vi "Compute Transfer Rate for FPGA.vi"(6 "Duty Rate":u16, 7 "Clock Rate (minus 1)":u16) -> (2 "Current Value":u16, 3 "Output":bool)   [LabVIEW 2013]
doc: "This SubVI uses a counter to create a boolean output based upon the requested number of clock cycles and a duty cycle."
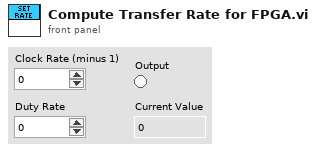
[diagram p1: front panel]
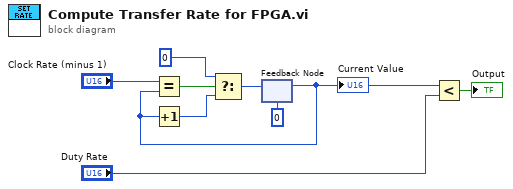
[diagram p0: block diagram]
diagram:
  n1 = feedback #1(u16 0) -> (w4:u16)
  "Current Value" <- w4
  n2 = Equal?(x="Clock Rate (minus 1)", y=w4) -> (x = y?=w7:bool)
  n3 = Increment(x=w4) -> (x+1=w5:u16)
  n4 = Select(t=u16 0, s=w7, f=w5) -> (s? t:f=w8:u16)
  n5 = feedback-in #1(w8) -> ()
  n6 = Less?(x=w4, y="Duty Rate") -> (x < y?=→"Output":bool)
